vi "波形发生器.vi"(2 "sampling info":cluster{"Fs":dbl, "#s":dbl}={"Fs"=1000.0, "#s"=1000.0} caption="采样信息" {"Fs" format="%.2p"}, 3 "formula":string="sin(w*t)*sin(2*pi(1)*t)" caption="公式", 4 "信噪比":dbl, 5 "square wave duty cycle (%)":dbl=50.0 caption="方波占空比(%)" format="%0.2f", 6 "phase":dbl caption="相位" format="%.2p", 7 "amplitude":dbl=1.0 caption="幅值" format="%0.2p", 8 "frequency":dbl=10.0 caption="频率" format="%0.2p", 9 "停止":bool, 10 "噪声选择":enum16{"高斯白噪声", "均匀白噪声", "无"}(ring), 11 "波形选择":enum16{"公式波", "三角波", "方波", "正弦波"}(ring)) -> (1 "波形图":waveform(dbl)(graph))   [LabVIEW 2017]
uses:
  <vilib>/measure/NI_MABase.lvlib
  <vilib>/measure/NI_MAPro.lvlib
panel:
  # "波 形 发 生 器"
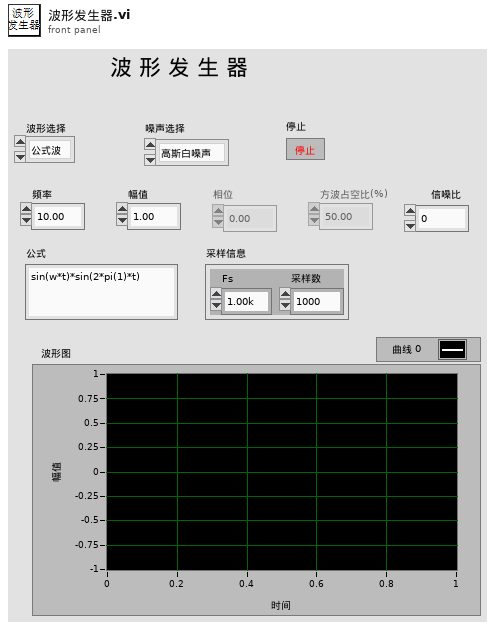
[diagram p1: front panel]
types:
  T1 = enum8{"Enabled", "Disabled", "Disabled and Grayed Out"}
  T2 = enum16{"Sine Wave", "Triangle Wave", "Square Wave", "Sawtooth Wave"}
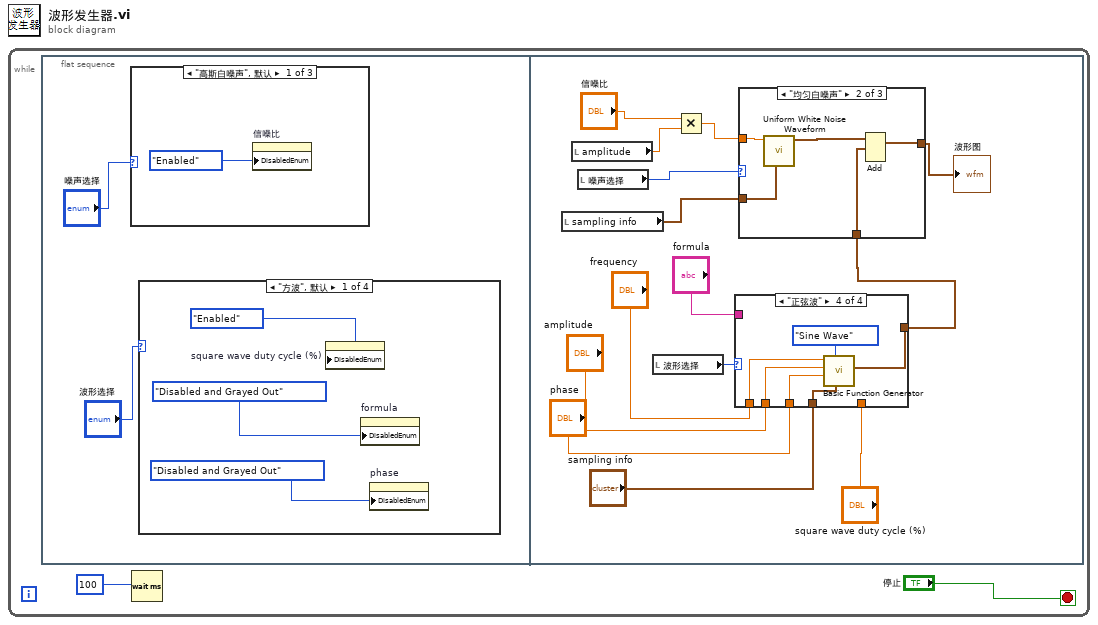
[diagram p0: block diagram]
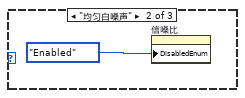
[diagram p2: hidden frame]
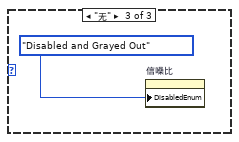
[diagram p3: hidden frame]
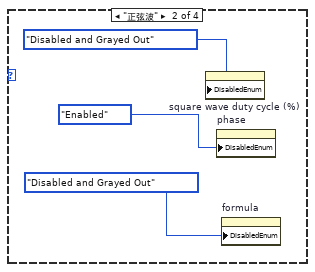
[diagram p4: hidden frame]
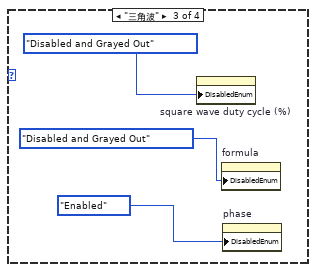
[diagram p5: hidden frame]
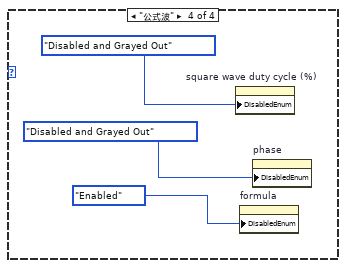
[diagram p6: hidden frame]
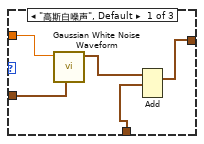
[diagram p7: hidden frame]
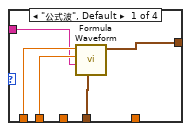
[diagram p9: hidden frame]
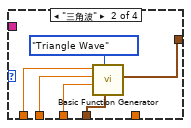
[diagram p10: hidden frame]
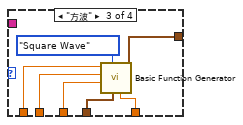
[diagram p11: hidden frame]
diagram:
  n1 = while {
    stop <- "停止" stop-if-true
    n2 = flat-sequence {
      frame #0 {
        n3 = case shown="\"高斯白噪声\", 默认" "噪声选择" {
          frame "高斯白噪声", Default {
            n4 = property on="信噪比" class="DigNum (严格)"("DisabledEnum"=T1."Enabled" ("禁用")) -> ()  [unwired: 2 in, 2 out]
          }
          frame "均匀白噪声" {
            n5 = property on="信噪比" class="DigNum (严格)"("DisabledEnum"=T1."Enabled" ("禁用")) -> ()  [unwired: 2 in, 2 out]
          }
          frame "无" {
            n6 = property on="信噪比" class="DigNum (严格)"("DisabledEnum"=T1."Disabled and Grayed Out" ("禁用")) -> ()  [unwired: 2 in, 2 out]
          }
        }
        n7 = case shown="\"方波\", 默认" "波形选择" {
          frame "方波", Default {
            n8 = property on="square wave duty cycle (%)" class="DigNum (严格)"("DisabledEnum"=T1."Enabled" ("禁用")) -> ()  [unwired: 2 in, 2 out]
            n9 = property on="formula" class="Str"("DisabledEnum"=T1."Disabled and Grayed Out" ("禁用")) -> ()  [unwired: 2 in, 2 out]
            n10 = property on="phase" class="DigNum (严格)"("DisabledEnum"=T1."Disabled and Grayed Out" ("禁用")) -> ()  [unwired: 2 in, 2 out]
          }
          frame "正弦波" {
            n11 = property on="square wave duty cycle (%)" class="DigNum (严格)"("DisabledEnum"=T1."Disabled and Grayed Out" ("禁用")) -> ()  [unwired: 2 in, 2 out]
            n12 = property on="phase" class="DigNum (严格)"("DisabledEnum"=T1."Enabled" ("禁用")) -> ()  [unwired: 2 in, 2 out]
            n13 = property on="formula" class="Str"("DisabledEnum"=T1."Disabled and Grayed Out" ("禁用")) -> ()  [unwired: 2 in, 2 out]
          }
          frame "三角波" {
            n14 = property on="square wave duty cycle (%)" class="DigNum (严格)"("DisabledEnum"=T1."Disabled and Grayed Out" ("禁用")) -> ()  [unwired: 2 in, 2 out]
            n15 = property on="formula" class="Str"("DisabledEnum"=T1."Disabled and Grayed Out" ("禁用")) -> ()  [unwired: 2 in, 2 out]
            n16 = property on="phase" class="DigNum (严格)"("DisabledEnum"=T1."Enabled" ("禁用")) -> ()  [unwired: 2 in, 2 out]
          }
          frame "公式波" {
            n17 = property on="square wave duty cycle (%)" class="DigNum (严格)"("DisabledEnum"=T1."Disabled and Grayed Out" ("禁用")) -> ()  [unwired: 2 in, 2 out]
            n18 = property on="formula" class="Str"("DisabledEnum"=T1."Enabled" ("禁用")) -> ()  [unwired: 2 in, 2 out]
            n19 = property on="phase" class="DigNum (严格)"("DisabledEnum"=T1."Disabled and Grayed Out" ("禁用")) -> ()  [unwired: 2 in, 2 out]
          }
        }
      }
      frame #1 {
        n20 = local read "sampling info"() -> (w22:cluster{"Fs":dbl, "#s":dbl})
        n21 = local read "amplitude"() -> (w24:dbl)
        n22 = local read "噪声选择"() -> (w26:enum16{"高斯白噪声", "均匀白噪声", "无"})
        n23 = local read "波形选择"() -> (w33:enum16{"公式波", "三角波", "方波", "正弦波"})
        n24 = Multiply(x="信噪比", y=w24) -> (x*y=w23:dbl)
        n25 = case shown="\"正弦波\"" w33 {
          tunnel: "frequency" -> [w49 w54 w61 w67]
          tunnel: "amplitude" -> [w48 w53 w60 w66]
          tunnel: "phase" -> [_ w52 w59 w65]
          tunnel: "sampling info" -> [w47 w51 w58 w64]
          tunnel: "square wave duty cycle (%)" -> [_ _ w57 _]
          tunnel: "formula" -> [w46 _ _ _]
          tunnel: [w45 w50 w56 w63] -> w21
          frame "公式波", Default {
            n26 = call <vilib>:"Formula Waveform.vi"("sampling info"=w47, "formula"=w46, "amplitude"=w48, "frequency"=w49) -> ("signal out"=w45:waveform(dbl))  [unwired: 6 in, 1 out]
          }
          frame "三角波" {
            n27 = call <vilib>:"Basic Function Generator.vi"("sampling info"=w51, "signal type"=T2."Triangle Wave", "phase"=w52, "amplitude"=w53, "frequency"=w54) -> ("signal out"=w50:waveform(dbl))  [unwired: 4 in, 2 out]
          }
          frame "方波" {
            n28 = call <vilib>:"Basic Function Generator.vi"("square wave duty cycle (%)"=w57, "sampling info"=w58, "signal type"=T2."Square Wave", "phase"=w59, "amplitude"=w60, "frequency"=w61) -> ("signal out"=w56:waveform(dbl))  [unwired: 3 in, 2 out]
          }
          frame "正弦波" {
            n29 = call <vilib>:"Basic Function Generator.vi"("sampling info"=w64, "signal type"=T2."Sine Wave", "phase"=w65, "amplitude"=w66, "frequency"=w67) -> ("signal out"=w63:waveform(dbl))  [unwired: 4 in, 2 out]
          }
        }
        n30 = case shown="\"均匀白噪声\"" w26 {
          tunnel: w23 -> [w38 w43 _]
          tunnel: w22 -> [w37 w42 _]
          tunnel: w21 -> [w35 w41 w44]
          tunnel: [w34 w39 w44] -> w20
          frame "高斯白噪声", Default {
            n31 = call <vilib>:"Gaussian White Noise Waveform.vi"("sampling info"=w37, "standard deviation"=w38) -> ("signal out"=w36:waveform(dbl))  [unwired: 8 in, 1 out]
            n32 = Add(1:w35, 2:w36) -> (0:w34:waveform(dbl))  [unwired: 1 in, 1 out]
          }
          frame "均匀白噪声" {
            n33 = call <vilib>:"Uniform White Noise Waveform.vi"("sampling info"=w42, "amplitude"=w43) -> ("signal out"=w40:waveform(dbl))  [unwired: 8 in, 1 out]
            n34 = Add(1:w41, 2:w40) -> (0:w39:waveform(dbl))  [unwired: 1 in, 1 out]
          }
          frame "无" {
          }
        }
        "波形图" <- w20
      }
    }
    n35 = Wait (ms)(milliseconds to wait=u32 100 ("毫秒计时值")) -> ()  [unwired: 1 out]
  }
